vi "find_sync_begin.vi"(0 "Buffer":string) -> (1 "Found":bool, 2 "Buffer Out":string)   [LabVIEW 2022 SP3]
panel:
  in  "Sync Begin":u8=146
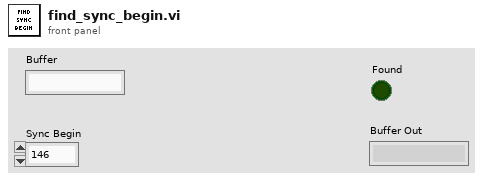
[diagram p1: front panel]
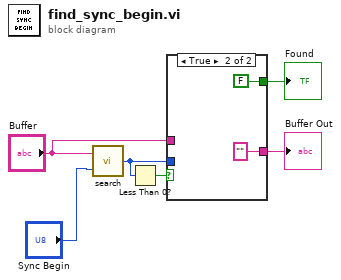
[diagram p0: block diagram]
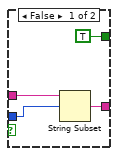
[diagram p2: hidden frame]
diagram:
  n1 = call "search.vi"("Byte"="Sync Begin", "Buffer"="Buffer") -> ("Index"=w2:i32)
  n2 = Less Than 0?(x=w2) -> (x < 0?=w6:bool)
  n3 = case shown="True" w6 {
    tunnel: [w9 ""] -> w5
    tunnel: [TRUE FALSE] -> w4
    tunnel: "Buffer" -> [w10 _]
    tunnel: w2 -> [w7 _]
    frame False {
      n4 = String Subset(string=w10, offset (0)=w7) -> (substring=w9:string)  [unwired: 1 in]
    }
    frame True {
    }
  }
  "Found" <- w4
  "Buffer Out" <- w5
